vi "Read callback UE.vi"(8 "error in (no error)":errorcluster, 11 "RocketPlotHandle in":refnum<class "RocketPlotHandle.lvclass">) -> (0 "error out":errorcluster, 2 "callback UE":refnum<user-event>, 3 "RocketPlotHandle out":refnum<class "RocketPlotHandle.lvclass">)   [LabVIEW 2021, in "RocketPlotHandle.lvclass"]
uses:
  RocketPlotHandle.lvclass
  RocketPlotHandle.lvclass/RocketPlotHandle.ctl
  SubVIs/callback type.ctl
  SubVIs/callback data.ctl
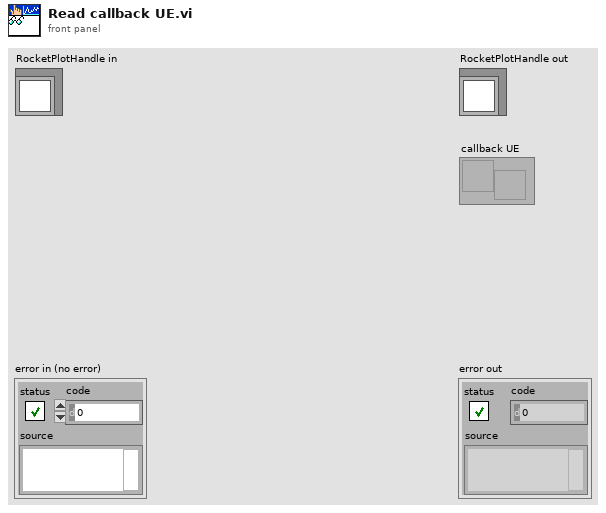
[diagram p1: front panel]
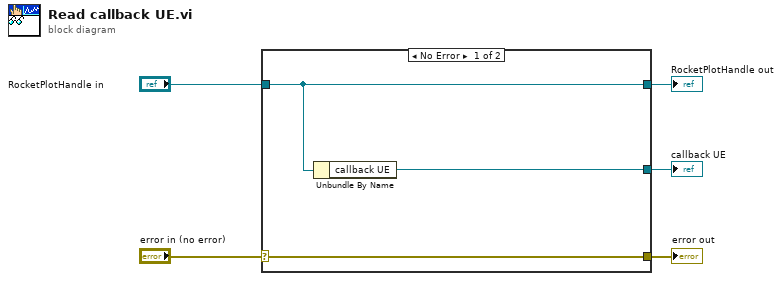
[diagram p0: block diagram]
diagram:
  n1 = case shown="No Error" "error in (no error)" {
    selector: "error in (no error)" -> [w8 w9]
    tunnel: [w8 w9] -> w4
    tunnel: [w7 w10] -> w2
    tunnel: "RocketPlotHandle in" -> [w7 w10]
    tunnel: [w6 _] -> w1
    frame No Error {
      n2 = Unbundle By Name(w7) -> ("callback UE"=w6:refnum<user-event>)
    }
    frame Error {
    }
  }
  "error out" <- w4
  "RocketPlotHandle out" <- w2
  "callback UE" <- w1
